vi "iSPIM_Device.vi"(7 "Device-specific in":variant, 8 "error in (no error)":errorcluster, 10 "Position in":dbl[](array[numeric]), 11 "Operation":T2(ring)) -> (0 "error out":errorcluster, 1 "Device properties":cluster{"Axes":string[], "Tolerance":dbl[][]}, 2 "Position out":dbl[](array[numeric]), 3 "Status":T1, 5 "Device-specific out":variant)   [LabVIEW 2015]
uses:
  <vilib>/DAQmx/write.llb/DAQmx Write (Analog 2D DBL NChan NSamp).vi
  <vilib>/DAQmx/create/channels.llb/DAQmx Create Channel (AO-Voltage-Basic).vi
  <vilib>/DAQmx/miscellaneous.llb/DAQmx Fill In Error Info.vi
  <resource>/objmgr/daqmx.rc
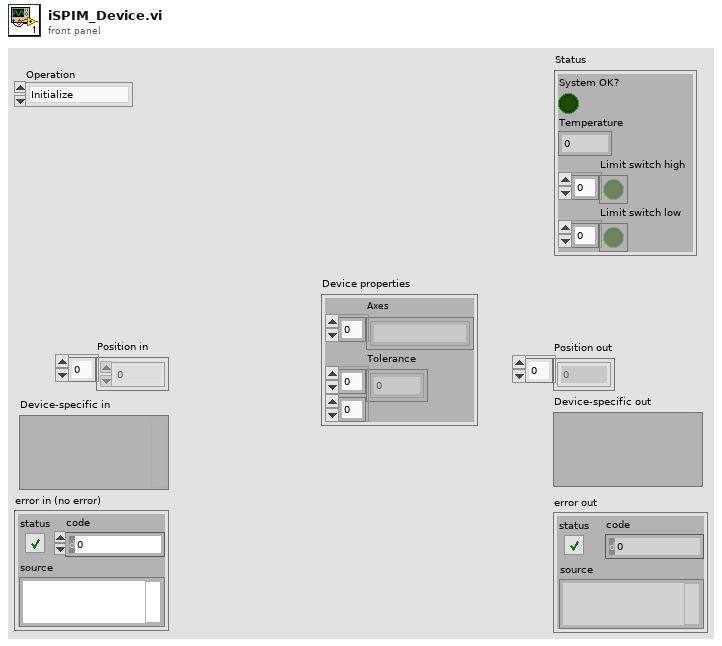
[diagram p1: front panel]
types:
  T1 = cluster{"System OK?":bool, "Temperature":dbl, "Limit switch high":bool[], "Limit switch low":bool[]}
  T2 = enum16{"Initialize", "Shut down", "Set position", "Get position", "Get status", "Other settings"}
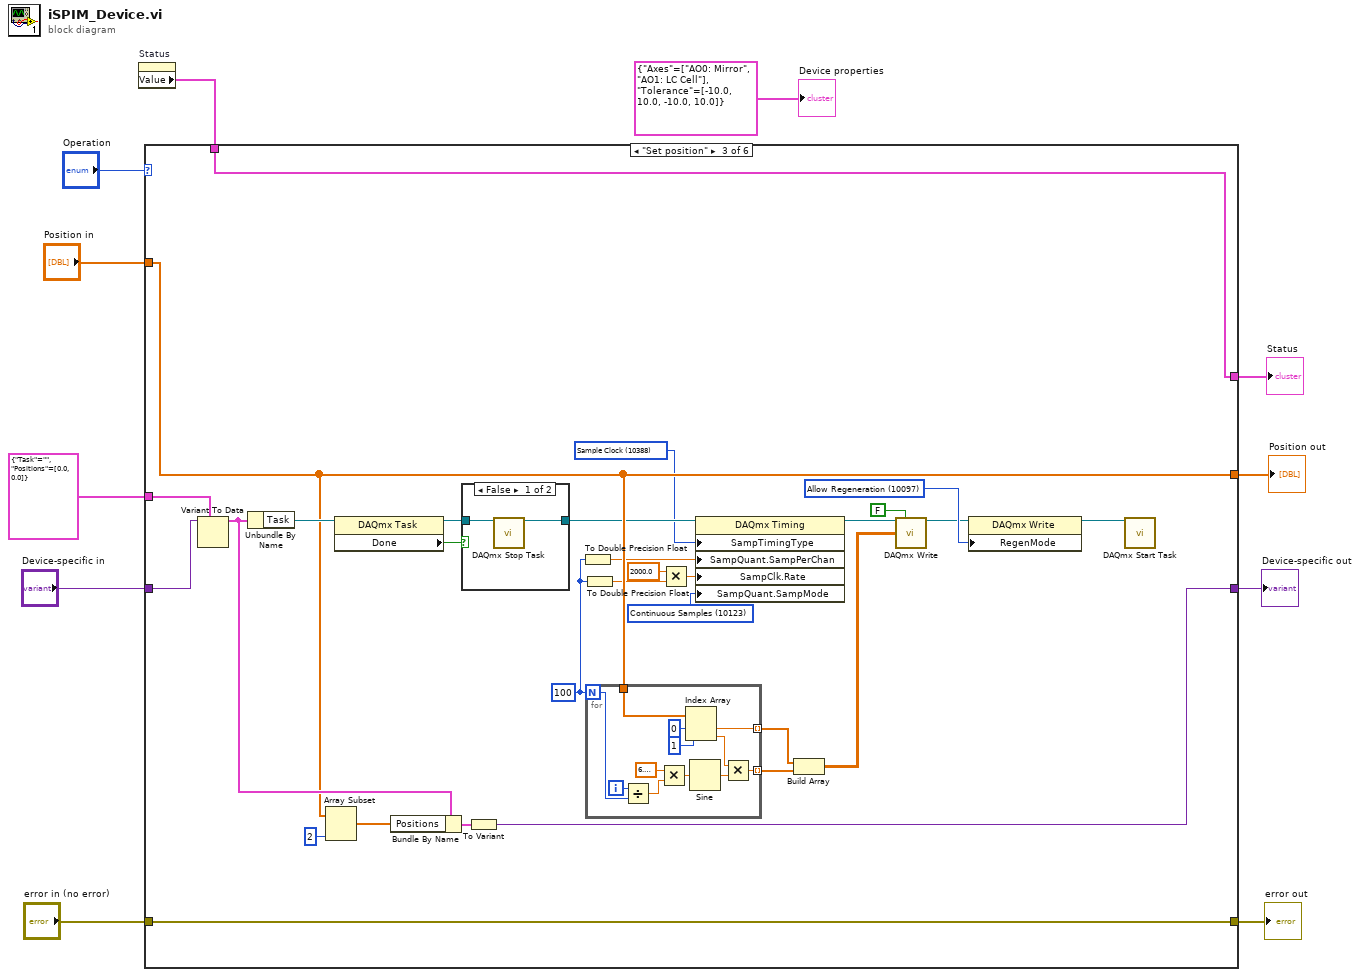
[diagram p0: block diagram]
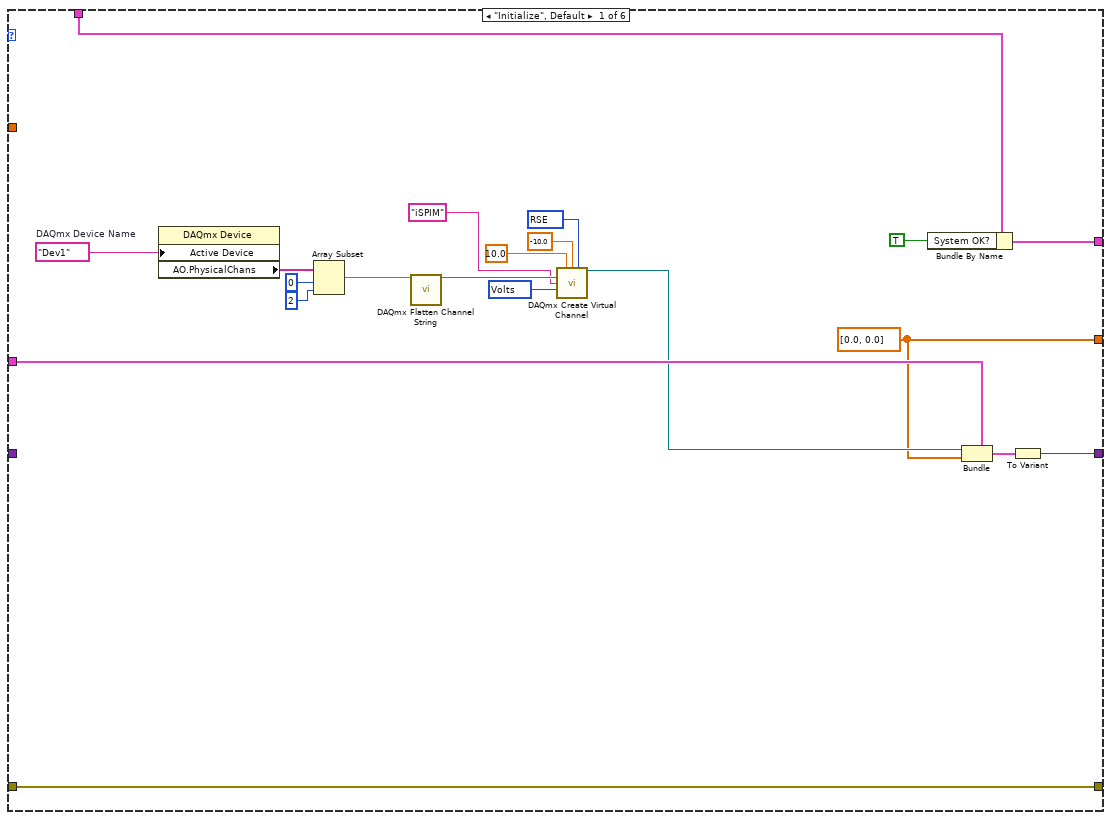
[diagram p2: hidden frame]
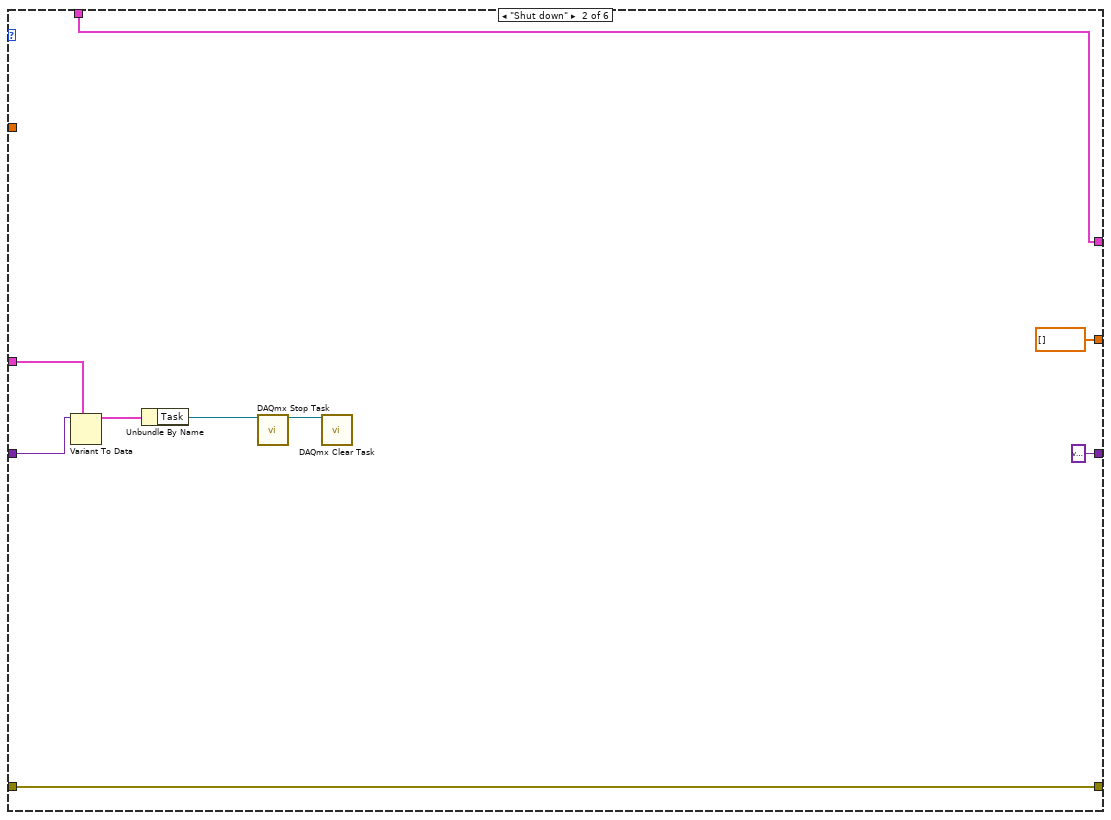
[diagram p3: hidden frame]
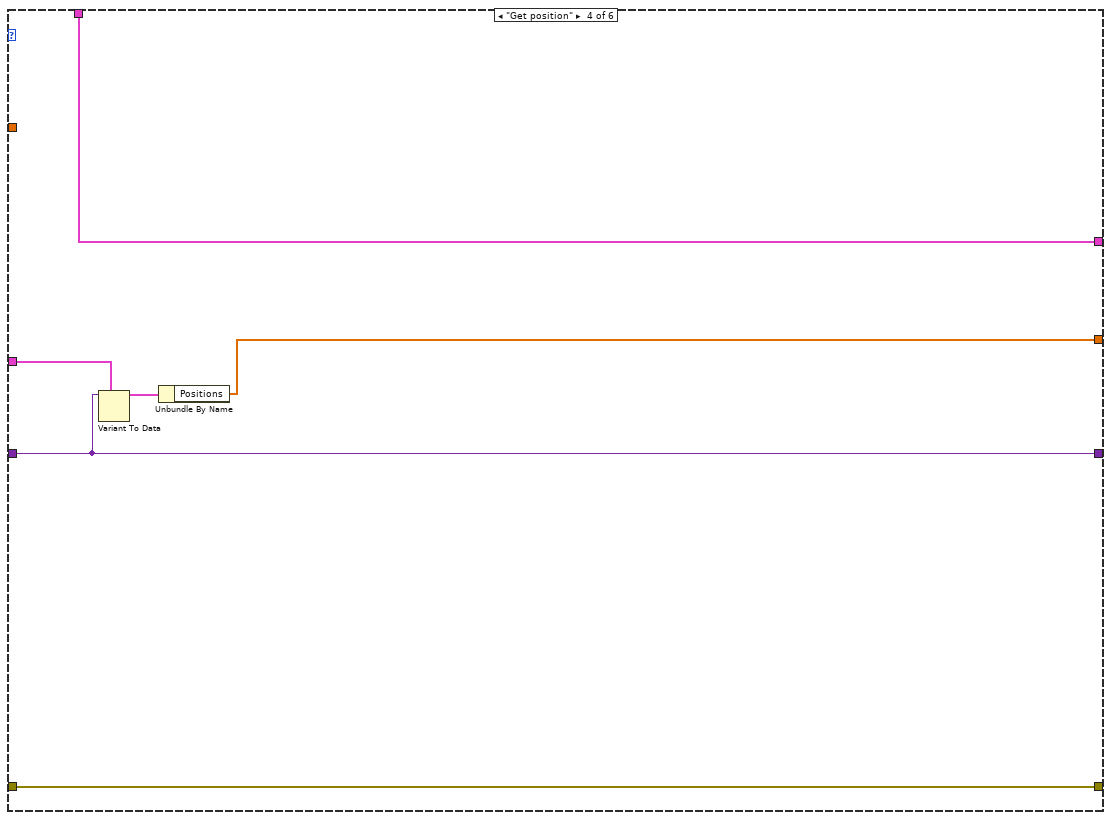
[diagram p5: hidden frame]
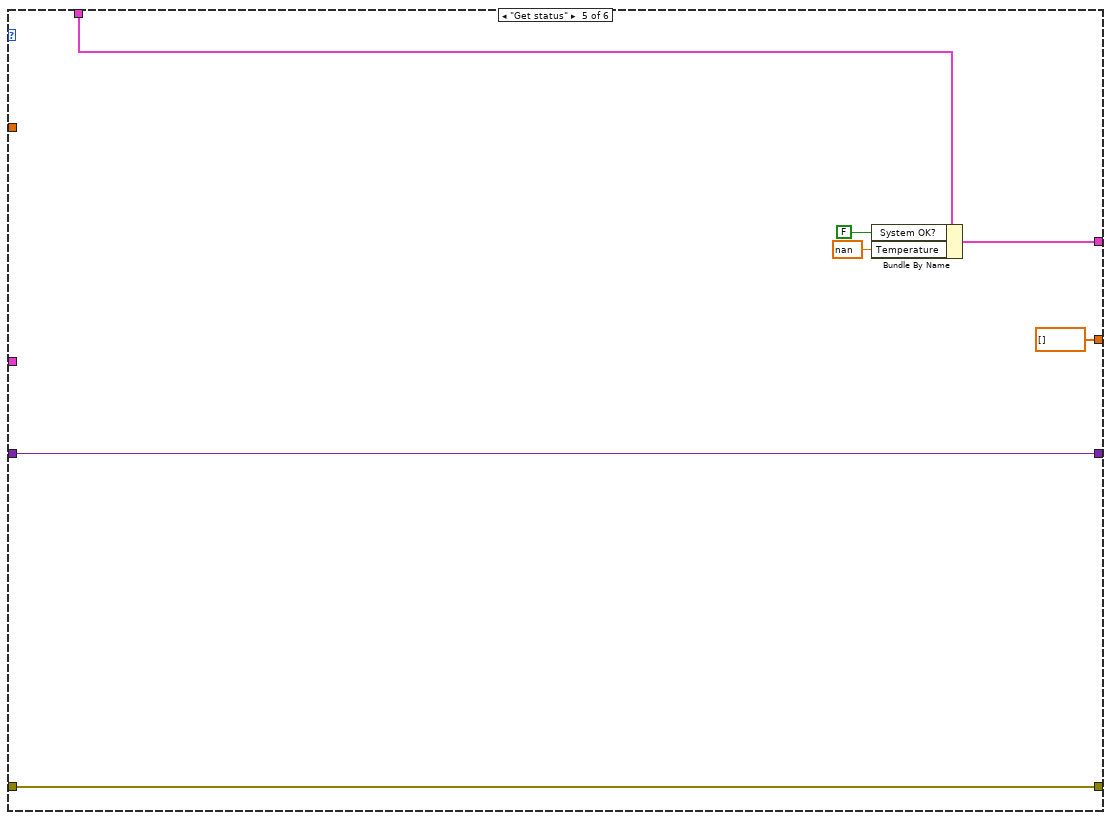
[diagram p6: hidden frame]
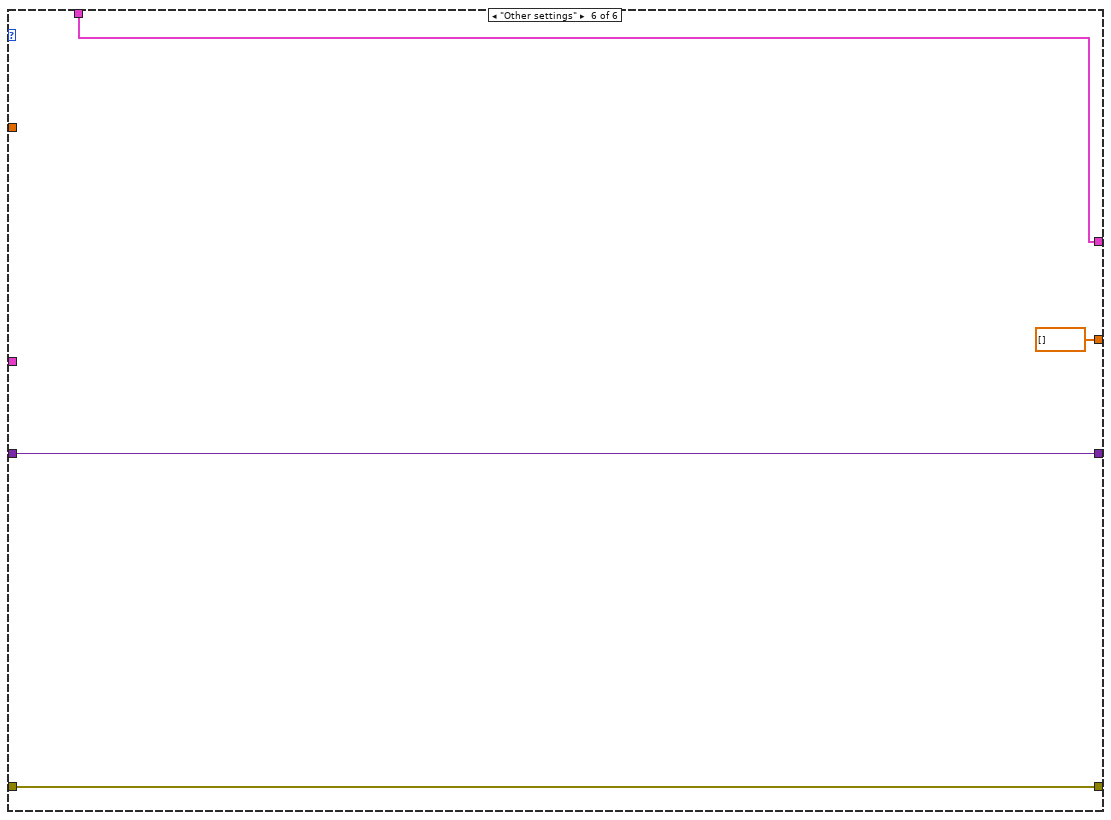
[diagram p7: hidden frame]
diagram:
  n1 = property on="Status" class="Clust (strict)"() -> ("Value"=w10:T1)  [unwired: 2 in, 2 out]
  n2 = case shown="\"Set position\"" "Operation" {
    tunnel: "Position in" -> [_ _ w57 _ _ _]
    tunnel: w10 -> [w31 w40 w69 w90 w97 w101]
    tunnel: [w30 w40 w69 w90 w96 w101] -> w9
    tunnel: "Device-specific in" -> [_ w37 w66 w88 w93 w100]
    tunnel: [w13 dbl[] [] ("Position in") w57 w85 dbl[] [] ("Position in") dbl[] [] ("Position in")] -> w6
    tunnel: [w16 variant ("Device-specific in") w53 w88 w93 w100] -> w5
    tunnel: [w28 w39 w68 w89 w92 w99] -> w4
    tunnel: "error in (no error)" -> [w28 w39 w68 w89 w92 w99]
    tunnel: cluster{"Task":refnum<k21>, "Positions":dbl[]} {"Task"="", "Positions"=[0.0, 0.0]} -> [w15 w36 w67 w87 _ _]
    frame "Initialize", Default {
      w18 = 10348 items=["Volts"=10348, "From Custom Scale"=10065] ("units")
      w21 = 10083 items=["Default"=-1, "RSE"=10083, "Differential"=10106, "Pseudodifferential"=12529] ("output terminal configuration")
      w27 = tag "Dev1"  # DAQmx Device Name
      w13 = dbl[] [0.0, 0.0] ("Position in")
      n3 = property class="DAQmx Device"("Active Device"=w27) -> ("AO.PhysicalChans"=w26:tag[])  [unwired: 2 in, 2 out]
      n4 = Array Subset(array=w26, index=0, length=2 ("index")) -> (w23:tag[])
      n5 = call <vilib>:"DAQmx Flatten Channel String.vi"("names in"=w23) -> ("names out"=w22:string)  [unwired: 13 in, 1 out]
      n6 = call-poly <vilib>:"DAQmx Create Virtual Channel.vi"("maximum value"=10.0, "minimum value"=-10.0, "output terminal configuration"=w21, "physical channels"=w22, "name to assign"="iSPIM", "units"=w18) -> ("task out"=w14:refnum<k21>)  [unwired: 8 in, 1 out]
      n7 = Bundle By Name(cluster=w31, "System OK?"=TRUE) -> (w30:T1)
      n8 = Bundle(cluster=w15, "Task"=w14, "Positions"=w13) -> (w12:cluster{"Task":refnum<k21>, "Positions":dbl[]})
      n9 = To Variant(anything=w12) -> (Variant=w16:variant)
    }
    frame "Shut down" {
      n10 = Variant To Data(type=w36, Variant=w37) -> (data=w35:cluster{"Task":refnum<k21>, "Positions":dbl[]})  [unwired: 1 in, 1 out]
      n11 = Unbundle By Name(w35) -> ("Task"=w32:refnum<k21>)
      n12 = call <vilib>:"DAQmx Stop Task.vi"("task/channels in"=w32) -> ("task out"=w34:refnum<k21>)  [unwired: 13 in, 1 out]
      n13 = call <vilib>:"DAQmx Clear Task.vi"("task in"=w34) -> ()  [unwired: 14 in, 1 out]
    }
    frame "Set position" {
      w41 = 10388 items=["Sample Clock"=10388, "Burst Handshake"=12548, "Handshake"=10389, "Implicit"=10451, "On Demand"=10390, "Change Detection"=12504, "Pipelined Sample Clock"=14668] ("SampTimingType")
      w46 = 10097 items=["Allow Regeneration"=10097, "Do Not Allow Regeneration"=10158] ("RegenMode")
      w62 = 10123 items=["Finite Samples"=10178, "Continuous Samples"=10123, "Hardware Timed Single Point"=12522] ("SampQuant.SampMode")
      w51 = 100
      n14 = Variant To Data(type=w67, Variant=w66) -> (data=w58:cluster{"Task":refnum<k21>, "Positions":dbl[]})  [unwired: 1 in, 1 out]
      n15 = Unbundle By Name(w58) -> ("Task"=w59:refnum<k21>)
      n16 = Array Subset(array=w57, length=2) -> (w55:dbl[])  [unwired: 1 in]
      n17 = property class="DAQmx Task"(reference=w59) -> (reference out=w61:refnum<k21>, "Done"=w60:bool)  [unwired: 1 in, 1 out]
      n18 = Bundle By Name(cluster=w58, "Positions"=w55) -> (w54:cluster{"Task":refnum<k21>, "Positions":dbl[]})
      n19 = case shown="False" w60 {
        tunnel: [w71 w72] -> w45
        tunnel: w61 -> [w70 w72]
        frame False {
          n20 = call <vilib>:"DAQmx Stop Task.vi"("task/channels in"=w70) -> ("task out"=w71:refnum<k21>)  [unwired: 13 in, 1 out]
        }
        frame True {
        }
      }
      n21 = To Variant(anything=w54) -> (Variant=w53:variant)
      n22 = To Double Precision Float(number=w51) -> (double precision float=w50:dbl)
      n23 = To Double Precision Float(number=w51) -> (double precision float=w49:dbl)
      n24 = for {
        N: w51 -> [w74]
        tunnel: w57 -> [w84]
        tunnel: [w81] -> w47 mode=indexing
        tunnel: [w77] -> w48 mode=indexing
        i -> [w73]
        n25 = Divide(x=w73, y=w74) -> (x/y=w78:dbl)
        n26 = Multiply(x=6.283185307179586, y=w78) -> (x*y=w80:dbl)
        n27 = Index Array(array=w84, index #1=0 ("index"), index #2=1 ("index")) -> (element #1=w81:dbl, element #2=w75:dbl)
        n28 = Sine(x=w80) -> (sin(x)=w76:dbl)
        n29 = Multiply(x=w75, y=w76) -> (x*y=w77:dbl)
      }
      n30 = Multiply(x=2000.0, y=w49) -> (x*y=w64:dbl)
      n31 = property class="DAQmx Timing"(reference=w45, "SampTimingType"=w41, "SampQuant.SampPerChan"=w50, "SampClk.Rate"=w64, "SampQuant.SampMode"=w62) -> (reference out=w65:refnum<k21>)  [unwired: 1 in, 1 out]
      n32 = Build Array(w47, w48) -> (w52:dbl[][])
      n33 = call-poly <vilib>:"DAQmx Write.vi"("task/channels in"=w65, "auto start"=FALSE, "data"=w52) -> ("task out"=w44:refnum<k21>)  [unwired: 10 in, 2 out]
      n34 = property class="DAQmx Write"(reference=w44, "RegenMode"=w46) -> (reference out=w42:refnum<k21>)  [unwired: 1 in, 1 out]
      n35 = call <vilib>:"DAQmx Start Task.vi"("task/channels in"=w42) -> ()  [unwired: 13 in, 2 out]
    }
    frame "Get position" {
      n36 = Variant To Data(type=w87, Variant=w88) -> (data=w86:cluster{"Task":refnum<k21>, "Positions":dbl[]})  [unwired: 1 in, 1 out]
      n37 = Unbundle By Name(w86) -> ("Positions"=w85:dbl[])
    }
    frame "Get status" {
      n38 = Bundle By Name(cluster=w97, "System OK?"=FALSE, "Temperature"=nan) -> (w96:T1)
    }
    frame "Other settings" {
    }
  }
  "Status" <- w9
  "Device-specific out" <- w5
  "error out" <- w4
  "Position out" <- w6
  "Device properties" <- cluster{"Axes":string[], "Tolerance":dbl[][]} {"Axes"=["AO0: Mirror", "AO1: LC Cell"], "Tolerance"=[[-10.0, 10.0], [-10.0, 10.0]]} ("Device properties")
